vi "Module.Init Working Dirs - Old.vi"(7 "Public Docs":bool, 8 "error in":errorcluster, 11 "App Name":string) -> (0 "error out":errorcluster, 3 "Working Dirs":T1)   [LabVIEW 2016, in "KATE_Lib.lvlib" / "Module Utils.lvlib"]
uses:
  Module Utils.lvlib
  Module.Working Dirs.ctl
  <vilib>/Utility/sysdir.llb/System Directory Type.ctl
  <vilib>/Utility/config.llb/Read Key (Path).vi
  <vilib>/Utility/config.llb/NI_LVConfig.lvlib
  Files/File Utils.lvlib
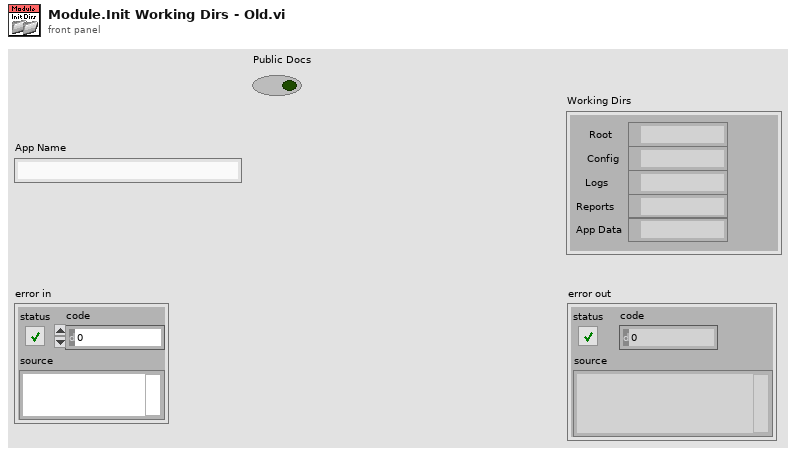
[diagram p1: front panel]
types:
  T1 = typedef "KATE_Lib.lvlib/Module Utils.lvlib/Module.Working Dirs.ctl" = cluster{"Root":path, "Config":path, "Logs":path, "Reports":path, "App Data":path}
  T2 = typedef "System Directory Type.ctl" = i32
  T3 = typedef "NI_LVConfig.lvlib/Config Data RefNum.ctl" = refnum<k1>
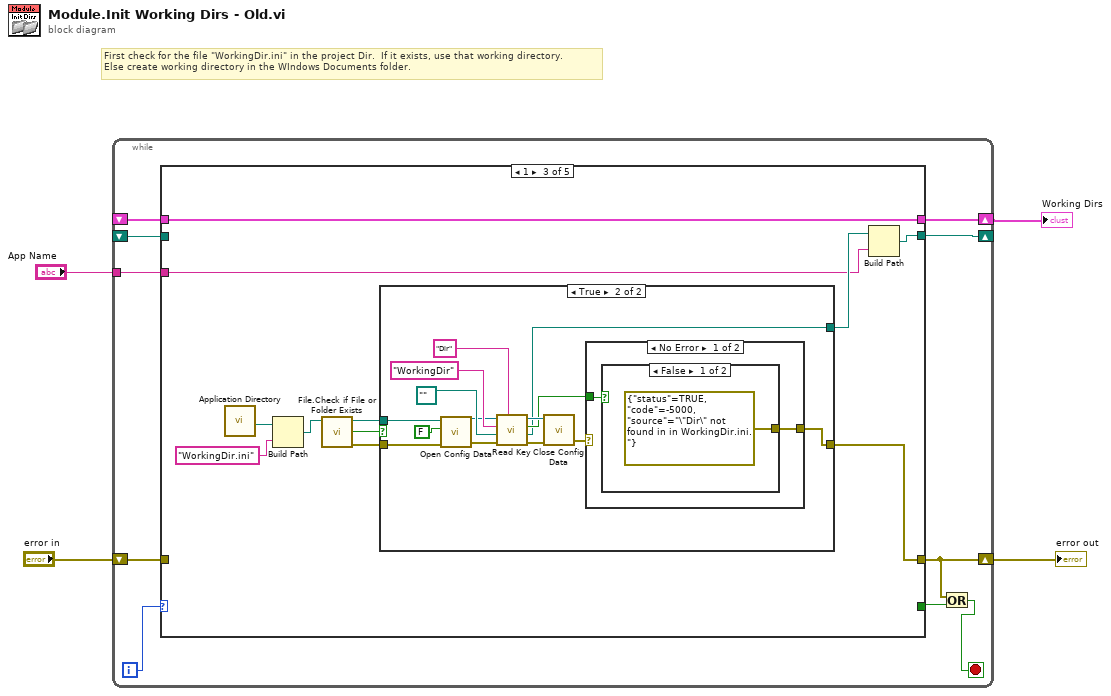
[diagram p0: block diagram]
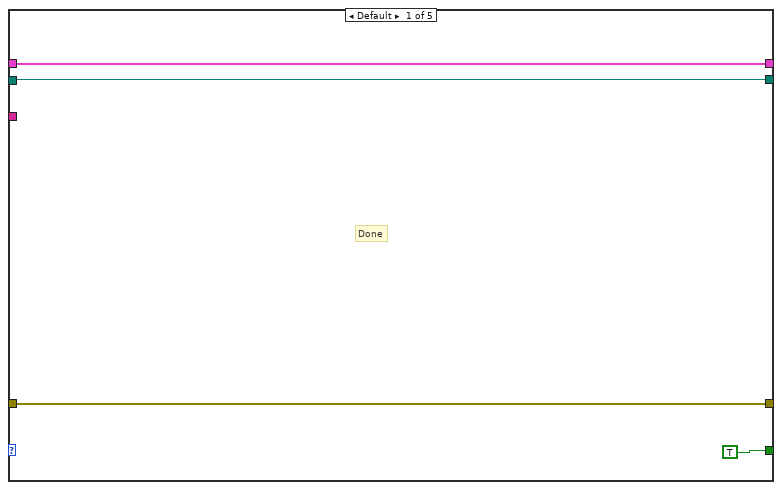
[diagram p2: hidden frame]
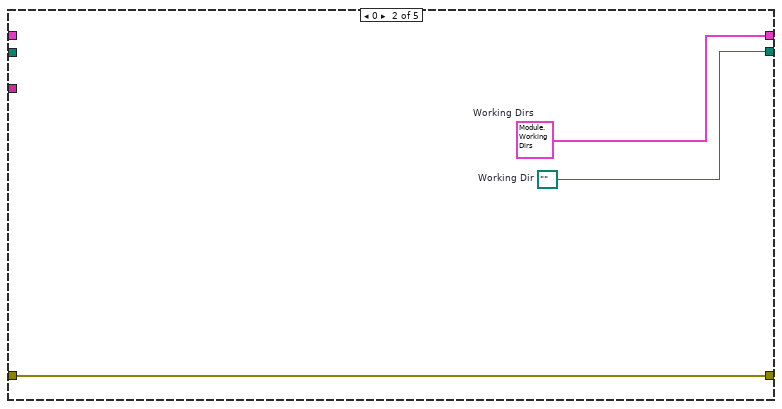
[diagram p3: hidden frame]
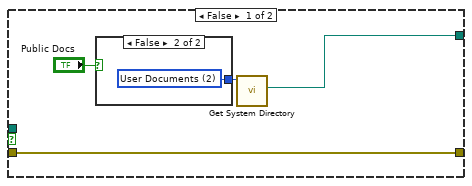
[diagram p4: hidden frame]
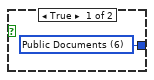
[diagram p5: hidden frame]
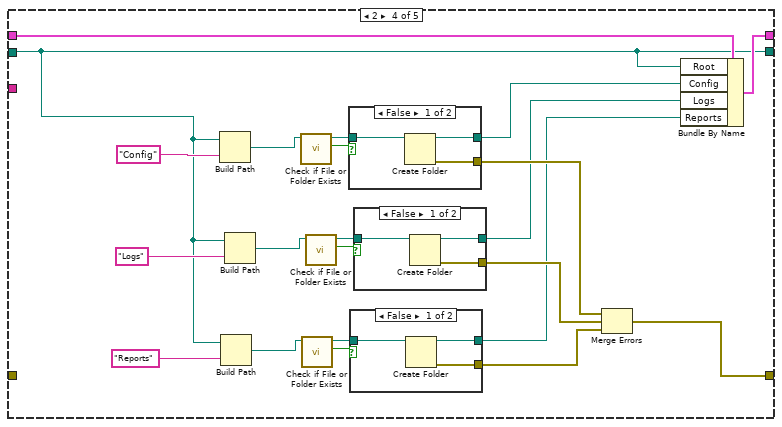
[diagram p8: hidden frame]
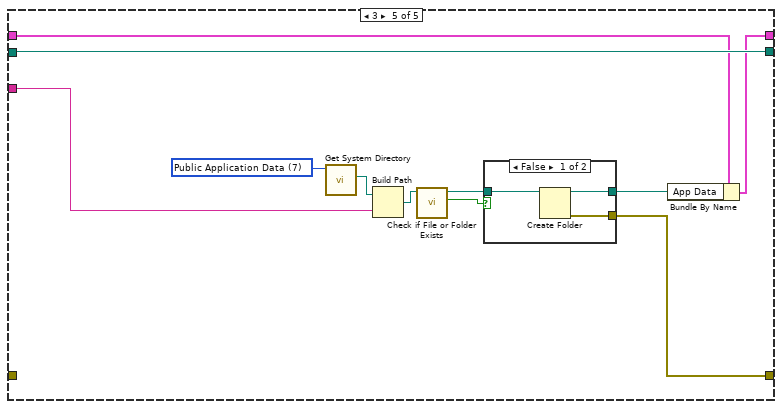
[diagram p12: hidden frame]
diagram:
  # "First check for the file \"WorkingDir.ini\" in the project Dir.  If it exists, use that working directory.\nElse create working directory in the WIndows Documents folder."
  n1 = while {
    shift-right: [w10] -> w3
    shift-left: "error in" -> [w13]
    shift-right: [w12] -> w1
    shift-left: _ -> [w7]
    tunnel: "App Name" -> [w8]
    shift-right: [w5] -> _
    shift-left: _ -> [w6]
    i -> [w14]
    stop <- w9 stop-if-true
    n2 = case shown="1" w14 {
      tunnel: [TRUE _ _ _ _] -> w11
      tunnel: [w17 w20 w28 w58 w95] -> w10
      tunnel: w13 -> [w17 w20 _ _ _]
      tunnel: [w16 w21 w29 w77 w92] -> w12
      tunnel: w8 -> [_ _ w23 _ w96]
      tunnel: w7 -> [w16 _ w29 w78 w93]
      tunnel: w6 -> [w15 _ _ w57 w94]
      tunnel: [w15 w19 w22 w57 w94] -> w5
      frame Default {
        # "Done"
      }
      frame 0 {
        w19 = path ""  # Working Dir
        w21 = T1 {"Root"=path "", "Config"=path "", "Logs"=path "", "Reports"=path "", "App Data"=path ""}  # Working Dirs
      }
      frame 1 {
        n3 = call <vilib>:"Application Directory.vi"() -> ("Application Directory"=w25:path)
        n4 = Build Path(base path=w25, name or relative path="WorkingDir.ini") -> (appended path=w27:path)
        n5 = call "File.Check if File or Folder Exists.vi"("Path"=w27) -> ("error out"=w31:errorcluster, "Exists"=w30:bool, "Dup Path"=w32:path)  [unwired: 7 in, 1 out]
        n6 = case shown="True" w30 {
          tunnel: w32 -> [_ w44]
          tunnel: w31 -> [w34 w43]
          tunnel: [w34 w40] -> w28
          tunnel: [w33 w39] -> w24
          frame False {
            n7 = case shown="False" "Public Docs" {
              tunnel: [w37 w38] -> w35
              frame True {
                w37 = T2 6 items=["User Home"=0, "User Desktop"=1, "User Documents"=2, "User Application Data"=3, "User Preferences"=4, "User Temporary"=5, "Public Documents"=6, "Public Application Data"=7, "Public Preferences"=8, "Public Cache"=13, "System Core Libraries"=9, "System Installed Libraries"=10, "Application Files"=11, "Boot Volume Root"=12] ("system directory type")
              }
              frame False {
                w38 = T2 2 items=["User Home"=0, "User Desktop"=1, "User Documents"=2, "User Application Data"=3, "User Preferences"=4, "User Temporary"=5, "Public Documents"=6, "Public Application Data"=7, "Public Preferences"=8, "Public Cache"=13, "System Core Libraries"=9, "System Installed Libraries"=10, "Application Files"=11, "Boot Volume Root"=12] ("system directory type")
              }
            }
            n8 = call <vilib>:"Get System Directory.vi"("system directory type"=w35) -> ("system directory"=w33:path)  [unwired: 10 in]
          }
          frame True {
            n9 = call <vilib>:"Open Config Data.vi"("error in (no error)"=w43, "create file if necessary (T)"=FALSE, "configuration file path"=w44) -> ("error out"=w47:errorcluster, "refnum"=w48:T3)  [unwired: 6 in, 1 out]
            n10 = call-poly <vilib>:"Read Key.vi"("section"="Dir", "error in (no error)"=w47, "default value"=path "" ("Working Dir"), "key"="WorkingDir", "refnum"=w48) -> ("error out"=w46:errorcluster, "value"=w39:path, "found?"=w41:bool, "refnum out"=w45:T3)  [unwired: 3 in]
            n11 = call <vilib>:"Close Config Data.vi"("error in (no error)"=w46, "refnum"=w45) -> ("error out"=w42:errorcluster)  [unwired: 8 in, 1 out]
            n12 = case shown="No Error" w42 {
              selector: w42 -> [_ w56]
              tunnel: w41 -> [w54 _]
              tunnel: [w53 w56] -> w40
              frame No Error {
                n13 = case shown="False" w54 {
                  tunnel: [errorcluster {"status"=TRUE, "code"=-5000, "source"="\"Dir\" not found in in WorkingDir.ini."} ("error constant") _] -> w53
                  frame False {
                  }
                  frame True {
                  }
                }
              }
              frame Error {
              }
            }
          }
        }
        n14 = Build Path(base path=w24, name or relative path=w23) -> (appended path=w22:path)
      }
      frame 2 {
        n15 = Build Path(base path=w57, name or relative path="Config") -> (appended path=w68:path)
        n16 = Build Path(base path=w57, name or relative path="Reports") -> (appended path=w66:path)
        n17 = Build Path(base path=w57, name or relative path="Logs") -> (appended path=w67:path)
        n18 = call <vilib>:"Check if File or Folder Exists.vi"("path"=w68) -> ("file or folder exists?"=w76:bool, "dup path"=w75:path)  [unwired: 8 in, 1 out]
        n19 = call <vilib>:"Check if File or Folder Exists.vi"("path"=w66) -> ("file or folder exists?"=w65:bool, "dup path"=w64:path)  [unwired: 8 in, 1 out]
        n20 = call <vilib>:"Check if File or Folder Exists.vi"("path"=w67) -> ("file or folder exists?"=w71:bool, "dup path"=w72:path)  [unwired: 8 in, 1 out]
        n21 = case shown="False" w76 {
          tunnel: [w89 _] -> w70
          tunnel: w75 -> [w88 w90]
          tunnel: [w87 w90] -> w62
          frame False {
            n22 = Create Folder(path (use dialog)=w88) -> (created path=w87:path, error out=w89:errorcluster)  [unwired: 2 in, 1 out]
          }
          frame True {
          }
        }
        n23 = case shown="False" w65 {
          tunnel: [w81 _] -> w59
          tunnel: w64 -> [w80 w82]
          tunnel: [w79 w82] -> w60
          frame False {
            n24 = Create Folder(path (use dialog)=w80) -> (created path=w79:path, error out=w81:errorcluster)  [unwired: 2 in, 1 out]
          }
          frame True {
          }
        }
        n25 = case shown="False" w71 {
          tunnel: [w85 _] -> w69
          tunnel: w72 -> [w84 w86]
          tunnel: [w83 w86] -> w61
          frame False {
            n26 = Create Folder(path (use dialog)=w84) -> (created path=w83:path, error out=w85:errorcluster)  [unwired: 2 in, 1 out]
          }
          frame True {
          }
        }
        n27 = Merge Errors(w70, w69, w59) -> (w58:errorcluster)
        n28 = Bundle By Name(cluster=w78, "Root"=w57, "Config"=w62, "Logs"=w61, "Reports"=w60) -> (w77:T1)
      }
      frame 3 {
        w100 = T2 7 items=["User Home"=0, "User Desktop"=1, "User Documents"=2, "User Application Data"=3, "User Preferences"=4, "User Temporary"=5, "Public Documents"=6, "Public Application Data"=7, "Public Preferences"=8, "Public Cache"=13, "System Core Libraries"=9, "System Installed Libraries"=10, "Application Files"=11, "Boot Volume Root"=12] ("system directory type")
        n29 = call <vilib>:"Get System Directory.vi"("system directory type"=w100) -> ("system directory"=w101:path)  [unwired: 10 in]
        n30 = Build Path(base path=w101, name or relative path=w96) -> (appended path=w99:path)
        n31 = call <vilib>:"Check if File or Folder Exists.vi"("path"=w99) -> ("file or folder exists?"=w98:bool, "dup path"=w97:path)  [unwired: 8 in, 1 out]
        n32 = case shown="False" w98 {
          tunnel: [w104 _] -> w95
          tunnel: w97 -> [w103 w105]
          tunnel: [w102 w105] -> w91
          frame False {
            n33 = Create Folder(path (use dialog)=w103) -> (created path=w102:path, error out=w104:errorcluster)  [unwired: 2 in, 1 out]
          }
          frame True {
          }
        }
        n34 = Bundle By Name(cluster=w93, "App Data"=w91) -> (w92:T1)
      }
    }
    n35 = Or(x=w10, y=w11) -> (x .or. y?=w9:bool)
  }
  "Working Dirs" <- w1
  "error out" <- w3
